vi "Send Trigger and Wait for OPC.vi"(8 "error in":errorcluster {"code" format="%.0x"}, 10 "Timeout":u32=20000, 11 "Session In":refnum<visa-resource-name>="GPIB0::16::INSTR") -> (0 "error out":errorcluster {"code" format="%.0x"}, 2 "OPC?":string, 3 "Session Out":refnum<visa-resource-name>)   [LabVIEW 2018]
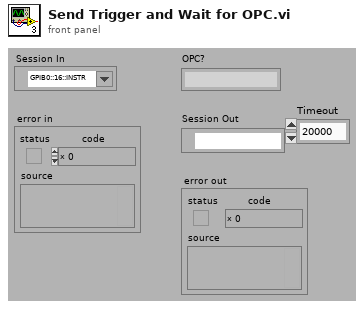
[diagram p1: front panel]
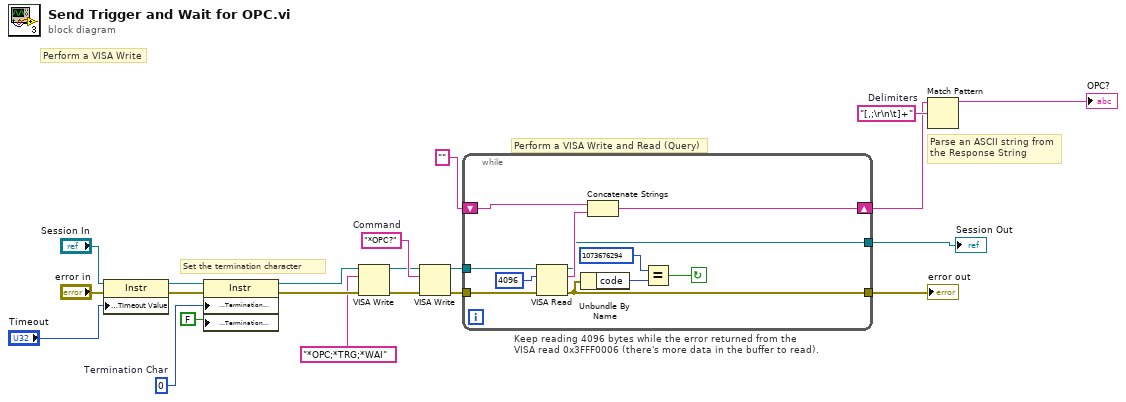
[diagram p0: block diagram]
diagram:
  w5 = "[,;\r\n\t]+"  # Delimiters
  w7 = "*OPC?"  # Command
  w16 = u8 0  # Termination Char
  # "Parse an ASCII string from the Response String"
  # "Perform a VISA Write and Read (Query)"
  # "Keep reading 4096 bytes while the error returned from the\nVISA read 0x3FFF0006 (there's more data in the buffer to read)."
  # "Perform a VISA Write"
  # "Set the termination character"
  n1 = property class="Instr"(reference="Session In", error in="error in", "General Settings:Timeout Value"="Timeout") -> (reference out=w15:refnum<visa-resource-name>, error out=w18:errorcluster)
  n2 = property class="Instr"(reference=w15, error in=w18, "Message Based Settings:Termination Character"=w16, "Message Based Settings:Termination Character Enable"=FALSE ("enable")) -> (reference out=w3:refnum<visa-resource-name>, error out=w17:errorcluster)
  n3 = VISA Write(VISA resource name=w3, write buffer="*OPC;*TRG;*WAI" ("StaticText"), error in (no error)=w17) -> (VISA resource name out=w2:refnum<visa-resource-name>, error out=w13:errorcluster)  [unwired: 1 out]
  n4 = VISA Write(VISA resource name=w2, write buffer=w7, error in (no error)=w13) -> (VISA resource name out=w11:refnum<visa-resource-name>, error out=w10:errorcluster)  [unwired: 1 out]
  n5 = while {
    tunnel: w11 -> [w29]
    shift-right: [w23] -> w4
    shift-left: "" -> [w28]
    tunnel: w10 -> [w26]
    tunnel: [w25] -> w9
    tunnel: [w22] -> w1
    stop <- w24 continue-if-true
    n6 = VISA Read(VISA resource name=w29, byte count=u32 4096 ("byte count (0)"), error in (no error)=w26) -> (VISA resource name out=w22:refnum<visa-resource-name>, read buffer=w27:string, error out=w25:errorcluster)  [unwired: 1 out]
    n7 = Unbundle By Name(w25) -> ("code"=w31:i32)
    n8 = Concatenate Strings(w28, w27) -> (w23:string)
    n9 = Equal?(x=1073676294, y=w31) -> (x = y?=w24:bool)
  }
  "error out" <- w9
  "Session Out" <- w1
  n10 = Match Pattern(string=w4, regular expression=w5) -> (before substring=→"OPC?":string)  [unwired: 4 out]
